vi "res_INT_offset.vi"(10 "ST_results_info":T1, 11 "INT_position":i32) -> (3 "results_byte_array_offset":i32)   [LabVIEW 2020]
uses:
  ST_results_info.ctl
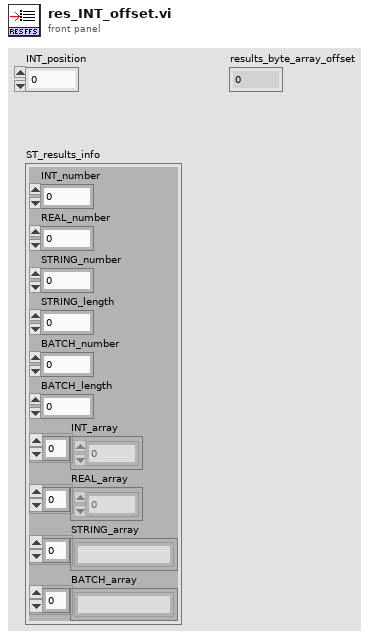
[diagram p1: front panel]
types:
  T1 = typedef "ST_results_info.ctl" = cluster{"INT_number":i32, "REAL_number":i32, "STRING_number":i32, "STRING_length":i32, "BATCH_number":i32, "BATCH_length":i32, "INT_array":i16[], "REAL_array":sgl[], "STRING_array":string[], "BATCH_array":string[]}
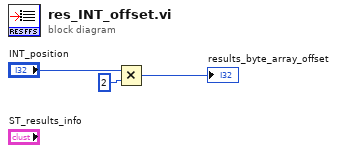
[diagram p0: block diagram]
diagram:
  n1 = Multiply(x="INT_position", y=2) -> (x*y=→"results_byte_array_offset":i32)
